vi "g.vi"() -> ()   [LabVIEW 2013]
panel:
  out "concatenated string":string
  out "error out 2":errorcluster
  out "VISA resource name out 2":refnum<visa-resource-name>
  in  "error in (no error) 2":errorcluster
  in  "VISA resource name 2":refnum<visa-resource-name>
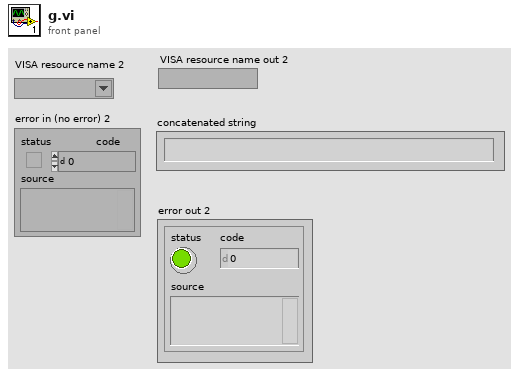
[diagram p1: front panel]
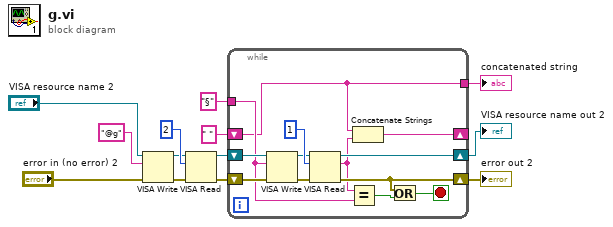
[diagram p0: block diagram]
diagram:
  n1 = VISA Write(VISA resource name="VISA resource name 2", write buffer="@g", error in (no error)="error in (no error) 2") -> (VISA resource name out=w9:refnum<visa-resource-name>, error out=w8:errorcluster)  [unwired: 1 out]
  n2 = VISA Read(VISA resource name=w9, byte count=u32 2, error in (no error)=w8) -> (VISA resource name out=w4:refnum<visa-resource-name>, error out=w3:errorcluster)  [unwired: 2 out]
  n3 = while {
    tunnel: "§" ("write buffer") -> [w17]
    shift-right: [w23] -> w6
    shift-left: w4 -> [w22]
    shift-right: [w19] -> w5
    shift-left: w3 -> [w21]
    shift-right: [w15] -> _
    shift-left: " " ("string") -> [w14]
    tunnel: [w14] -> w1
    stop <- w20 stop-if-true
    n4 = VISA Write(VISA resource name=w22, write buffer=w17, error in (no error)=w21) -> (VISA resource name out=w25:refnum<visa-resource-name>, error out=w24:errorcluster)  [unwired: 1 out]
    n5 = VISA Read(VISA resource name=w25, byte count=u32 1, error in (no error)=w24) -> (VISA resource name out=w23:refnum<visa-resource-name>, read buffer=w16:string, error out=w19:errorcluster)  [unwired: 1 out]
    n6 = Equal?(x=w16, y=w17) -> (x = y?=w18:bool)
    n7 = Concatenate Strings(w14, w16) -> (w15:string)
    n8 = Or(x=w19, y=w18) -> (x .or. y?=w20:bool)
  }
  "VISA resource name out 2" <- w6
  "error out 2" <- w5
  "concatenated string" <- w1
